vi "Check for Injector Timeout.vi"(8 "error in (no error)":errorcluster, 11 "Parameters":T1={"Name"="", "Rate.Hz"=0, "Injectors.Count"=0, "Injector.Timeout"=0.0, "Injector.Timer"=[], "Injector.Info"=[], "Events.Count"=[], "Event.Parameters"={"Shots"=0, "Shot.InitialVoltage"=0.0, "Shot.Stages"=0, "Stages"=[{"Stage.Dwell.Level"=0.0, "PullIn.Type"=enum."Pull In Transition Dwells", "PullIn.Level"=0.0, "Transition.Type"=enum."Stage Transition Voltage Level", "Transition.Level"=0.0}]}, "DMA.Ref"=refnum, "Waveform.Refs"=[], "Waveform.Sessions"=[], "Waveform.Enable"=refnum, "FPGA.Status"=refnum, "Search.Data"=refnum, "Results.Data"=refnum, "Results.Values"=[], "Results.Selections"=[]}) -> (0 "error out":errorcluster, 3 "Parameters":T1={"Name"="", "Rate.Hz"=0, "Injectors.Count"=0, "Injector.Timeout"=0.0, "Injector.Timer"=[], "Injector.Info"=[], "Events.Count"=[], "Event.Parameters"={"Shots"=0, "Shot.InitialVoltage"=0.0, "Shot.Stages"=0, "Stages"=[{"Stage.Dwell.Level"=0.0, "PullIn.Type"=enum."Pull In Transition Dwells", "PullIn.Level"=0.0, "Transition.Type"=enum."Stage Transition Voltage Level", "Transition.Level"=0.0}]}, "DMA.Ref"=refnum, "Waveform.Refs"=[], "Waveform.Sessions"=[], "Waveform.Enable"=refnum, "FPGA.Status"=refnum, "Search.Data"=refnum, "Results.Data"=refnum, "Results.Values"=[], "Results.Selections"=[]})   [LabVIEW 2015, in "Fuel Injector Analysis Addon Engine.lvlib"]
uses:
  Fuel Injector Analysis Addon Engine.lvlib
  Types/Async Parameters.ctl
  Shared/Types/Injector info.ctl
  Shared/Types/Shot.Parameters.ctl
  Shared/Types/Stage.Parameters.ctl
  Shared/Types/Stage.PullIn.Types.ctl
  Shared/Types/Stage.Transition.Types.ctl
  <vilib>/NI Veristand/Custom Device API/Waveform Data Reference.ctl
  <vilib>/NI VeriStand/Custom Device Waveform API/Single Waveform Write (DBL)/Single Waveform Write (DBL).lvclass
  <vilib>/NI/NIVS Inline Async API/_Data Access Engine/Data Access Engine/Types/Read.DVR.ctl
  <vilib>/NI/NIVS Inline Async API/_Data Access Engine/Access Type Classes/Read/Read.lvclass
  <vilib>/NI/NIVS Inline Async API/_Data Access Engine/Data Access Engine/Types/Write.DVR.ctl
  <vilib>/NI/NIVS Inline Async API/_Data Access Engine/Access Type Classes/Write/Write.lvclass
  Shared/Types/Analysis.Channels.Select.ctl
  <vilib>/NI/NIVS Inline Async API/_Data Access Engine/Access Type Classes/Write/Write.lvclass/Write.ctl
  <vilib>/NI/NIVS Inline Async API/_Data Access Engine/Data Access Engine/Methods/Write.Data.vi
  <vilib>/NI/NIVS Inline Async API/_Data Access Engine/Access Type Classes/Write/Write.ProcessData.vi
  <vilib>/NI/NIVS Inline Async API/_Data Access Engine/Data Access Engine/Data Access Engine.lvclass
  Shared/Fuel Injector Analysis Addon Shared.lvlib
  <vilib>/NI VeriStand/Custom Device API/Custom Device API.lvlib
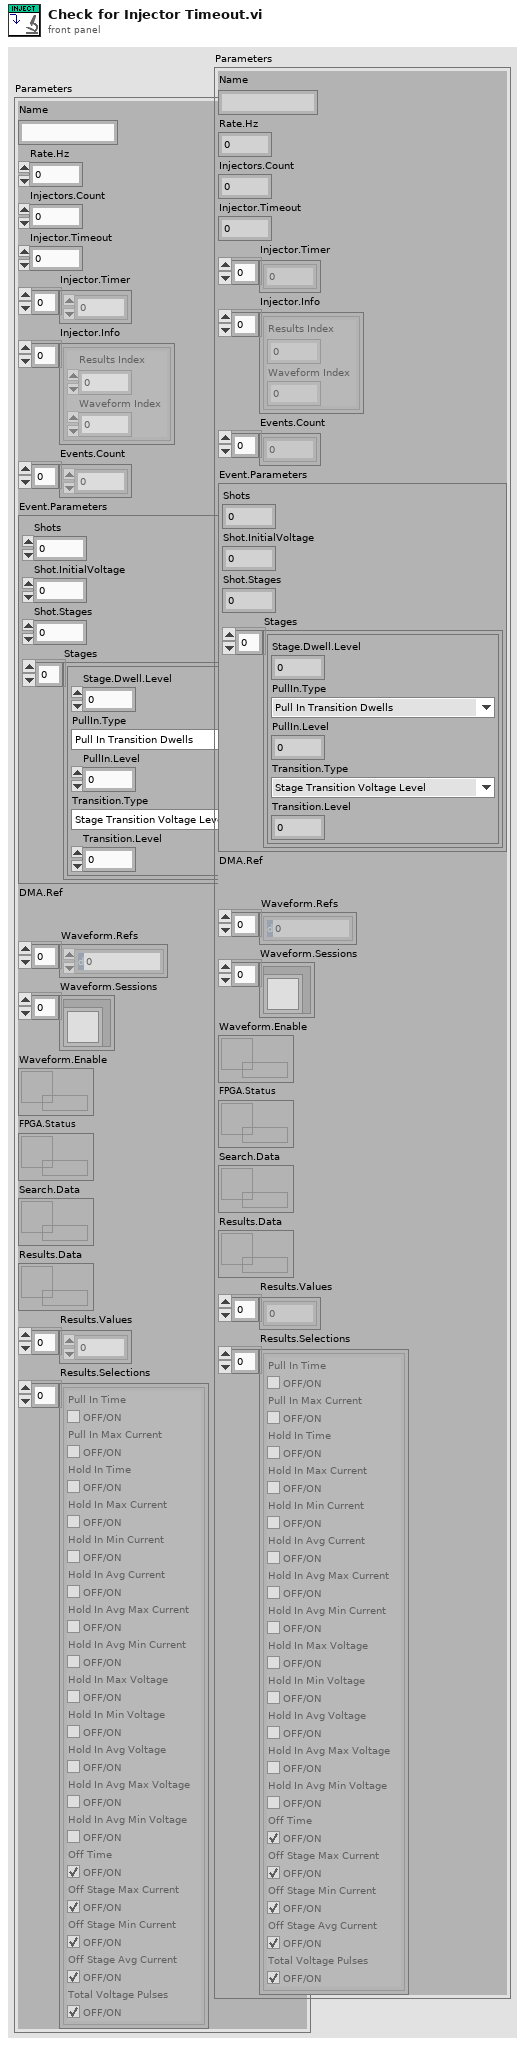
[diagram p1: front panel]
types:
  T1 = typedef "Fuel Injector Analysis Addon Engine.lvlib/Async Parameters.ctl" = cluster{"Name":string, "Rate.Hz":u32, "Injectors.Count":u8, "Injector.Timeout":dbl, "Injector.Timer":u32[], "Injector.Info":T2[], "Events.Count":u64[], "Event.Parameters":T3, "DMA.Ref":refnum<k20>, "Waveform.Refs":T7[], "Waveform.Sessions":refnum<class "Single Waveform Write (DBL).lvclass">[], "Waveform.Enable":T8, "FPGA.Status":T9, "Search.Data":T8, "Results.Data":T9, "Results.Values":dbl[], "Results.Selections":T10[]}
  T2 = typedef "Fuel Injector Analysis Addon Shared.lvlib/Injector info.ctl" = cluster{"Results Index":i32, "Waveform Index":i32}
  T3 = typedef "Fuel Injector Analysis Addon Shared.lvlib/Shot.Parameters.ctl" = cluster{"Shots":u32, "Shot.InitialVoltage":dbl, "Shot.Stages":u32, "Stages":T4[]}
  T4 = typedef "Fuel Injector Analysis Addon Shared.lvlib/Stage.Parameters.ctl" = cluster{"Stage.Dwell.Level":dbl, "PullIn.Type":T5, "PullIn.Level":dbl, "Transition.Type":T6, "Transition.Level":dbl}
  T5 = typedef "Fuel Injector Analysis Addon Shared.lvlib/Stage.PullIn.Types.ctl" = enum8{"Pull In Transition Dwells", "Pull In Transition Current Drop"}
  T6 = typedef "Fuel Injector Analysis Addon Shared.lvlib/Stage.Transition.Types.ctl" = enum8{"Stage Transition Dwell Time", "Stage Transition Voltage Level", "Stage Transition Current Drop"}
  T7 = typedef "Custom Device API.lvlib/Waveform Data Reference.ctl" = i32
  T8 = typedef "Data Access Engine.lvlib/Data Access Engine.lvclass/Read.DVR.ctl" = refnum<data-value>
  T9 = typedef "Data Access Engine.lvlib/Data Access Engine.lvclass/Write.DVR.ctl" = refnum<data-value>
  T10 = typedef "Fuel Injector Analysis Addon Shared.lvlib/Analysis.Channels.Select.ctl" = cluster{"Pull In Time":bool, "Pull In Max Current":bool, "Hold In Time":bool, "Hold In Max Current":bool, "Hold In Min Current":bool, "Hold In Avg Current":bool, "Hold In Avg Max Current":bool, "Hold In Avg Min Current":bool, "Hold In Max Voltage":bool, "Hold In Min Voltage":bool, "Hold In Avg Voltage":bool, "Hold In Avg Max Voltage":bool, "Hold In Avg Min Voltage":bool, "Off Time":bool, "Off Stage Max Current":bool, "Off Stage Min Current":bool, "Off Stage Avg Current":bool, "Total Voltage Pulses":bool}
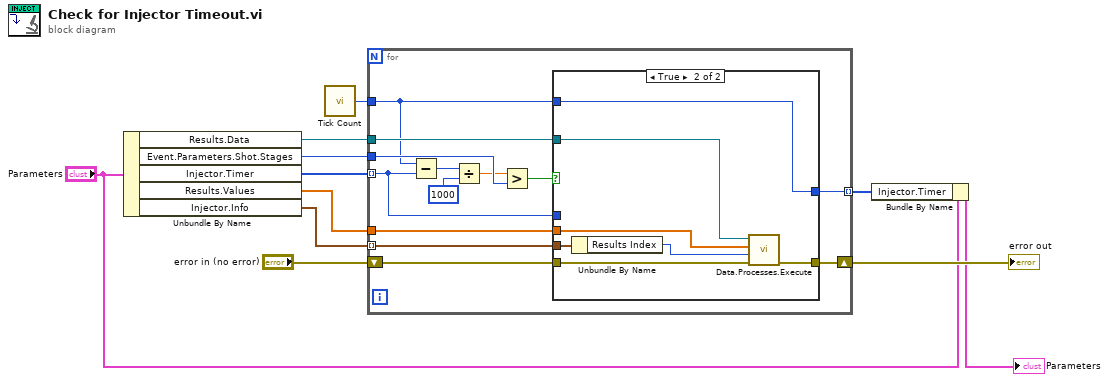
[diagram p0: block diagram]
diagram:
  n1 = Unbundle By Name("Parameters") -> ("Results.Data"=w6:T9, "Event.Parameters.Shot.Stages"=w7:u32, "Injector.Timer"=w8:u32[], "Results.Values"=w1:dbl[], "Injector.Info"=w5:T2[])
  n2 = call "Tick Count"() -> ("Tick Count(mSec)"=w9:u32)
  n3 = for {
    tunnel: w8 -> [w18] mode=indexing
    tunnel: w9 -> [w16]
    shift-right: [w13] -> w10
    shift-left: "error in (no error)" -> [w14]
    tunnel: w7 -> [w22]
    tunnel: w6 -> [w19]
    tunnel: [w17] -> w4 mode=indexing
    tunnel: w5 -> [w15] mode=indexing
    tunnel: w1 -> [w12]
    n4 = Subtract(x=w16, y=w18) -> (x-y=w24:u32)
    n5 = Divide(x=w24, y=u32 1000) -> (x/y=w21:dbl)
    n6 = Greater?(x=w21, y=w22) -> (0:w20:bool)
    n7 = case shown="True" w20 {
      tunnel: w19 -> [_ w32]
      tunnel: w18 -> [w26 _]
      tunnel: [w26 w33] -> w17
      tunnel: w16 -> [_ w33]
      tunnel: w15 -> [_ w29]
      tunnel: w14 -> [w25 w31]
      tunnel: [w25 w30] -> w13
      tunnel: w12 -> [_ w27]
      frame False {
      }
      frame True {
        n8 = Unbundle By Name(w29) -> ("Results Index"=w28:i32)
        n9 = call-poly <vilib>:"Data.Processes.Execute.vi"("error in (no error)"=w31, "Offset"=w28, "Values"=w27, "Ref"=w32) -> ("error out"=w30:errorcluster)  [unwired: 7 in]
      }
    }
  }
  "error out" <- w10
  n10 = Bundle By Name(cluster="Parameters", "Injector.Timer"=w4) -> (→"Parameters":T1)
